vi "Get Power Meter Default Value.vi"(0 "SG Path PM Accessor in":refnum<class "SG Path Simulated PM Accessor.lvclass">, 11 "error in":errorcluster) -> (4 "SG Path PM Accessor out":refnum<class "SG Path Simulated PM Accessor.lvclass">, 6 "Power Meter out":refnum<class "Power Meter Base.lvclass">, 15 "error out":errorcluster)   [LabVIEW 2023, in "RFFixtureCharact.Instruments.lvlib" / "SG Path Simulated PM Accessor.lvclass"]
uses:
  SG Path Simulated PM Accessor.lvclass
  Power Meter Base/Power Meter Base.lvclass
  Simulated/Simulated Power Meter.lvclass
  C:/srd-semi-rfcal-software/AuxTools/STSRFFixtureCharactUtility/Source/Code Modules/Fixture/Instruments/Power Meter/Power Meter Base/Power Meter Base.lvclass
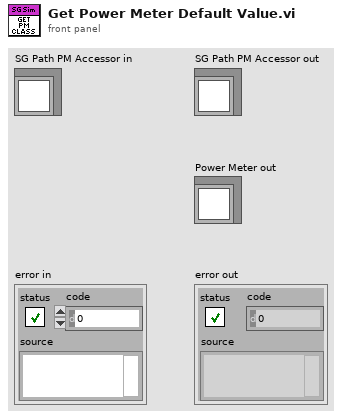
[diagram p1: front panel]
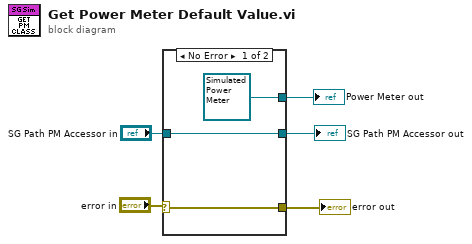
[diagram p0: block diagram]
diagram:
  n1 = case shown="No Error" "error in" {
    selector: "error in" -> [w7 w9]
    tunnel: [w8 w10] -> w4
    tunnel: "SG Path PM Accessor in" -> [w8 w10]
    tunnel: [w7 w9] -> w2
    tunnel: [refnum<class "Simulated Power Meter.lvclass"> refnum ("RFFixtureCharact.Scalar.lvlib:Simulated Power Meter.lvclass") _] -> w1
    frame No Error {
    }
    frame Error {
    }
  }
  "error out" <- w2
  "SG Path PM Accessor out" <- w4
  "Power Meter out" <- w1
